vi "add_data_line_exp.vi"(2 "error in (no error)":errorcluster, 3 "Array":dbl[](array[numeric]), 4 "Experiment.lvclass in":refnum<class "Experiment.lvclass">) -> (0 "error out":errorcluster, 1 "Experiment.lvclass out":refnum<class "Experiment.lvclass">)   [LabVIEW 2015, in "Experiment.lvclass"]
uses:
  Experiment.lvclass
  Experiment.lvclass/Experiment.ctl
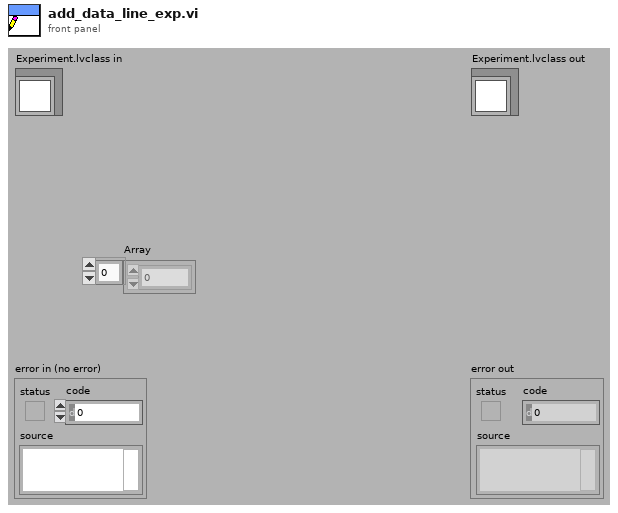
[diagram p1: front panel]
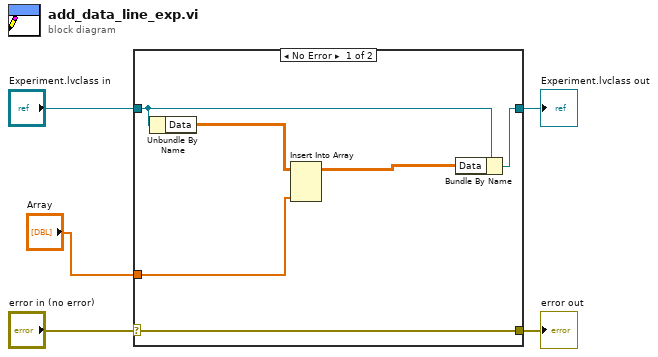
[diagram p0: block diagram]
diagram:
  n1 = case shown="No Error" "error in (no error)" {
    selector: "error in (no error)" -> [w11 w12]
    tunnel: [w11 w12] -> w4
    tunnel: [w10 w13] -> w2
    tunnel: "Experiment.lvclass in" -> [w6 w13]
    tunnel: "Array" -> [w7 _]
    frame No Error {
      n2 = Unbundle By Name(w6) -> ("Data"=w8:dbl[][])
      n3 = Insert Into Array(array=w8, new element=w7) -> (w9:dbl[][])  [unwired: 2 in]
      n4 = Bundle By Name(cluster=w6, "Data"=w9) -> (w10:refnum<class "Experiment.lvclass">)
    }
    frame Error {
    }
  }
  "error out" <- w4
  "Experiment.lvclass out" <- w2
